vi "Sum 3D [oxo] (DBL).vi"(1 "3D":dbl[][][](array[numeric])) -> (0 "2D":dbl[][](array[numeric]))   [LabVIEW 2009]
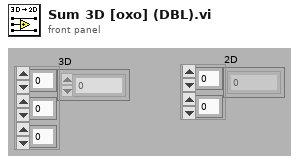
[diagram p1: front panel]
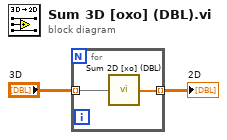
[diagram p0: block diagram]
diagram:
  n1 = for {
    tunnel: "3D" -> [w4] mode=indexing
    tunnel: [w3] -> w1 mode=indexing
    n2 = call "Sum 2D [xo] (DBL).vi"("2D"=w4) -> ("1D"=w3:dbl[])
  }
  "2D" <- w1
